vi "String to Hex.vi"(4 "Hex-like String":string) -> (1 "Hex String":string)   [LabVIEW 2015]
doc: "Classification: Unclassified\n\ntakes a hex-like string and turns it into a hex string\n\nby Jason Corwin"
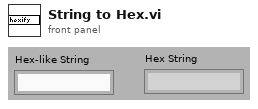
[diagram p1: front panel]
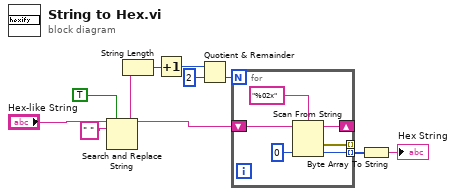
[diagram p0: block diagram]
diagram:
  n1 = Search and Replace String(replace all?=TRUE ("replace all? (F)"), input string="Hex-like String", search string=" ") -> (result string=w6:string)  [unwired: 5 in, 3 out]
  n2 = String Length(string=w6) -> (length=w2:i32)
  n3 = Increment(x=w2) -> (x+1=w1:i32)
  n4 = Quotient & Remainder(x=w1, y=2) -> (floor(x/y)=w3:i32)  [unwired: 1 out]
  n5 = for {
    N: w3 -> [_]
    shift-right: [w15] -> _
    shift-left: w6 -> [w16]
    tunnel: [w12] -> w7 mode=indexing
    tunnel: [w11] -> _ mode=indexing
    n6 = Scan From String(format string="%02x", input string=w16, default 1=u8 0 ("default value 1")) -> (remaining string=w15:string, error out=w11:errorcluster, output 1=w12:u8)  [unwired: 2 in, 1 out]
  }
  n7 = Byte Array To String(unsigned byte array=w7) -> (string=→"Hex String":string)
